vi "Dashboard Main.vi"() -> ()   [LabVIEW 2016]
uses:
  <vilib>/Utility/miscctls.llb/LVRowAndColumnTypeDef.ctl
  <vilib>/event_ctls.llb/eventvkey.ctl
  <vilib>/Rock Robotics/Network Tables/NT Read Numeric Array.vi
  Global 1.vi
  <vilib>/Rock Robotics/WPI/Dashboard/WPI_DashboardLogging Global.vi
  <vilib>/Rock Robotics/Network Tables/NT Read Boolean.vi
  <vilib>/Rock Robotics/Network Tables/NT Write Numeric Array.vi
panel:
  in  "TCP":refnum<k5>
  in  "Camera Settings Right":T1={"Frame Rate"=30, "Compression"=30, "Size"=1, "DB Camera Config"=FALSE} {"Frame Rate" scale=1.0..30.0; "Compression" scale=100.0..-1.0; "Size" items=["640x480", "320x240", "160x120"]}
  in  "Camera Name Right":string(combo)="No Camera Selection"
  out "Camera Info":cluster{"Mbps LED":bool, "Mbps":dbl, "fps":dbl} {"fps" format="%#.1g"; "Mbps" format="%#.1g"}
  in  "Camera Settings":T1={"Frame Rate"=30, "Compression"=30, "Size"=1, "DB Camera Config"=FALSE} {"Frame Rate" scale=1.0..30.0; "Compression" scale=100.0..-1.0; "Size" items=["640x480", "320x240", "160x120"]}
  in  "TCP":refnum<k5>
  in  "Rec Mode":enum32{"Stop", "Record", "Playback"}(radio)
  out "Robot IP":string
  out "Image Message":string="Timeout in Camera Communications"
  in  "Dashboard Tab":T2(tab)
  out "Boolean":bool
  in  "LockShooter":bool
  out "FrontShooter":dbl
  out "RearShooter":dbl
  in  "Select Auto":string(combo)="Select Autonomous ..."
  out "NT Connection":bool
  out "MotorChart R":cluster{"Numeric":dbl, "Numeric":dbl}(graph)
  out "MotorChart L":cluster{"Numeric":dbl, "Numeric":dbl}(graph)
  out "MotorSliders R":cluster{"MotorSlide1":dbl, "MotorSlide2":dbl} {"MotorSlide2" scale=-1.0..1.0 scale format="%#_2e"; "MotorSlide1" scale=-1.0..1.0 scale format="%#_2e"}
  out "MotorSliders L":cluster{"MotorSlide1":dbl, "MotorSlide2":dbl} {"MotorSlide2" scale=-1.0..1.0 scale format="%#_2e"; "MotorSlide1" scale=-1.0..1.0 scale format="%#_2e"}
  out "Gyro":dbl(knob) scale=0.0..360.0
  out "JS1 Z":dbl(slide) scale=-1.0..1.0 scale format="%#_2e"
  out "JS1 Graph":cluster{"X":dbl, "Y":dbl}[](graph)
  out "JS1 Buttons":T3
  out "JS2 Z":dbl(slide) scale=-1.0..1.0 scale format="%#_2e"
  out "JS2 Graph":cluster{"X":dbl, "Y":dbl}[](graph)
  out "JS2 Buttons":T3
  out "Mode":T4(ring)=enum."Auto Disabled"
  out "Camera Image Right":T5(plugin-control)
  in  "DB/String 9":string
  in  "DB/String 8":string
  in  "DB/String 7":string
  in  "DB/String 6":string
  in  "DB/String 5":string
  in  "DB/String 4":string
  in  "DB/String 3":string
  in  "DB/String 2":string
  in  "DB/String 1":string
  in  "DB/String 0":string
  in  "DB/Slider 0":dbl(slide) scale=0.0..5.0
  in  "DB/Slider 1":dbl(slide) scale=0.0..5.0
  in  "DB/Slider 2":dbl(slide) scale=0.0..5.0
  in  "DB/Slider 3":dbl(slide) scale=0.0..5.0
  out "DB/LED 3":bool
  out "DB/LED 2":bool
  out "DB/LED 1":bool
  out "DB/LED 0":bool
  in  "DB/Button 3":bool
  in  "DB/Button 2":bool
  in  "DB/Button 1":bool
  in  "DB/Button 0":bool caption="New Name"
  out "camera?":bool
  in  "dt":dbl
  out "TargetFound?":bool
  out "Yaw":dbl
  in  "AutonColor":string(combo)
  in  "AutonMode":string(combo)="DoNothing"
  out "AutonControl":string
  in  "PIDGains":dbl[](array[numeric])
  out "Countdown":sgl
  in  "Test Slider":dbl(slide) scale=0.0..100.0 scale format="%#_3g"
  in  "On/Off":bool caption="Solenoid"
  in  "Test Name":u16(ring) items=["Select the test to run..."]
  in  "Test Tree":string(tree)
  in  "Motor":cluster{"Value":dbl, "Enable":bool} {"Value" scale=-1.0..1.0 scale format="%#_3g"}
  out "Progress":T6 {"Test Progress" scale=0.0..100.0}
  in  "Rev/Fwd":cluster{"Forward":bool, "Reverse":bool}
  in  "Test Ring":u16(ring) items=["Monochrome", "Color"]
  out "Cmd Status":string
  in  "Execute Command":bool
  in  "Command Params":string[][](table)
  in  "Command Selection":i32(listbox)
  in  "CheckList":i32(listbox)
  out "Tree":string(tree)
  out "Camera Image":T5(plugin-control)
  out "Background":bool
  in  "Camera Name":string(combo)="No Camera Selection"
  # "HW"
  # "HW"
  # "Joysticks"
  # "Drive Motors"
  # "Front"
  # "Right"
  # "Left"
  # "Back"
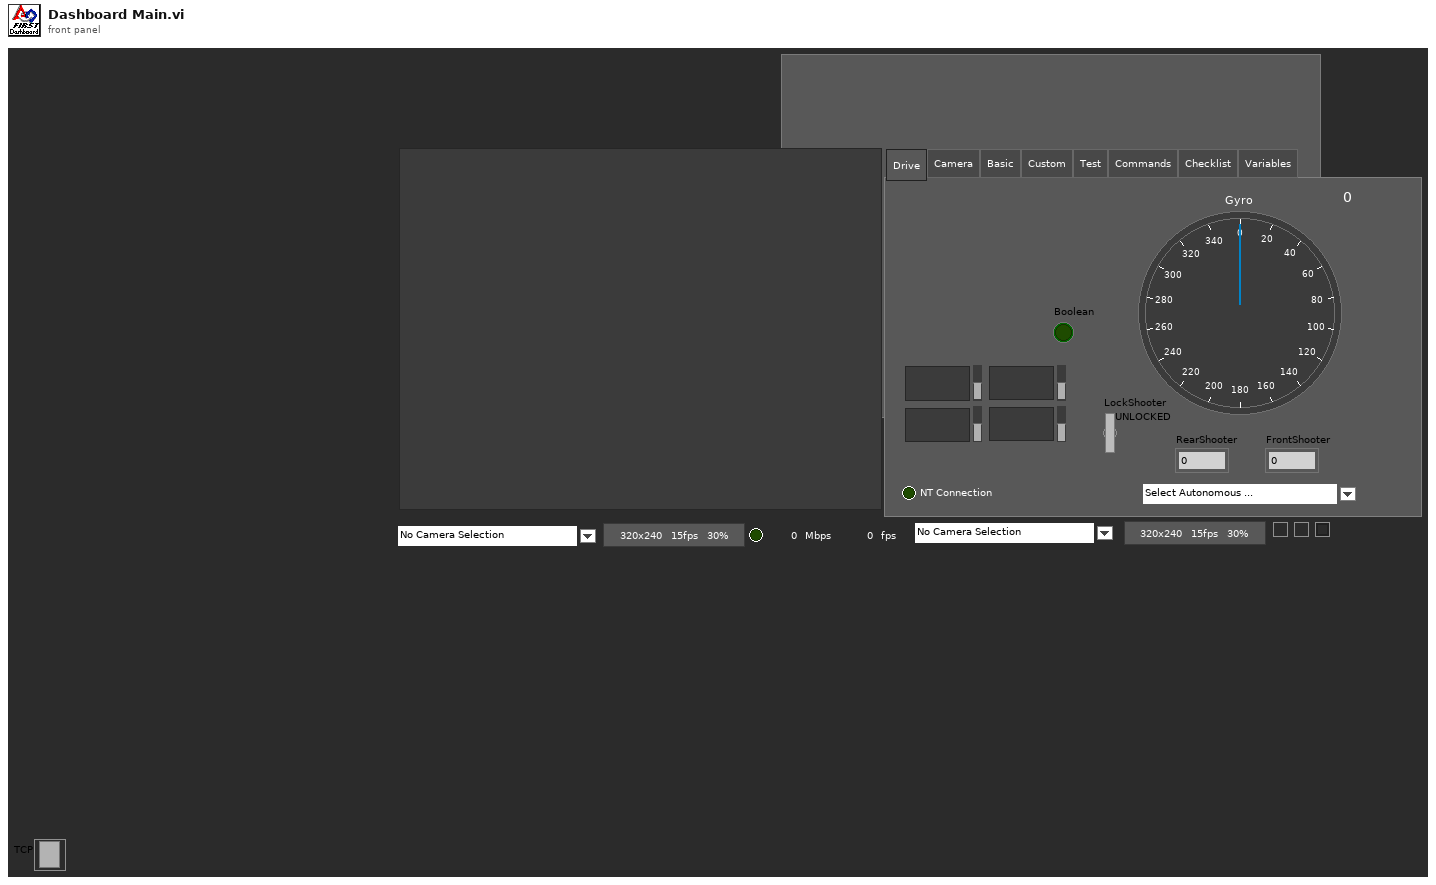
[diagram p1: front panel]
types:
  T1 = cluster{"Frame Rate":i32, "Compression":i32, "Size":u16, "DB Camera Config":bool}
  T2 = enum32{"Drive", "Camera", "Basic", "Custom", "Test", "Commands", "Checklist", "Variables"}
  T3 = cluster{bool, bool, bool, bool, bool, bool, bool, bool, bool, bool, bool, bool}
  T4 = enum8{"Tele-Op Disabled", "Tele-Op Enabled", "Auto Disabled", "Auto Enabled", "Test Disabled", "Test Enabled", "Disconnected", "No Code", "E-Stop"}
  T5 = typedef "IMAQ Image.ctl" = refnum<image>
  T6 = cluster{"Test Progress":u8, "Test Progress Text":string}
  T7 = typedef "Image Type" = u32
  T8 = cluster{"IDs":cluster{"RPC field ID":u16, "Unique ID":u16}, "String":string}
  T9 = enum32{"Drive", "Basic", "Custom", "Test", "Checklist", "Variables"}
  T10 = cluster{"Camera Image":refnum<vi>, "Dashboard Tab":refnum<vi>, "Background":refnum<vi>, "Rec Mode":refnum<vi>, "Test Slider":refnum<vi>, "On/Off ":refnum<vi>, "Test Ring":refnum<vi>, "Rev/Fwd":refnum<vi>, "Test Name":refnum<vi>, "Motor":refnum<vi>, "Progress":refnum<vi>, "CheckList":refnum<vi>, "Tree":refnum<vi>, "Test Tree":refnum<vi>, "Command Params":refnum<vi>, "Command Selection":refnum<vi>, "Execute Command":refnum<vi>, "Cmd Status":refnum<vi>, "Camera Settings":refnum<vi>, "Camera Name":refnum<vi>, "Camera Info":refnum<vi>, "Camera Settings Right":refnum<vi>, "Camera Name Right":refnum<vi>, "Camera Image Right":refnum<vi>}
  T11 = cluster{"Control Bits":cluster{"TestMode":bool, "Autonomous":bool, "Enabled":bool, "FMS Present":bool, bool, bool, bool, "E-Stop":bool}, "Team Station ":u8, "Countdown":sgl, "Joystick Values":cluster{"Axes":dbl[], "Buttons":bool[], "POVs":i16[]}[]}
  T12 = cluster{"Axes":dbl[], "Buttons":bool[], "POVs":i16[]}[]
  T13 = cluster{"Axes":dbl[], "Buttons":bool[], "POVs":i16[]}
  T14 = cluster{"Error Strings":string, "Disable Counts":cluster{u16, u16}, "Rail Faults":cluster{u16, u16, u16}, "Robot IP":string, "DB Mode":u8, "Event Info":cluster{"Name":string, "Type":u8, "Number":u16, "Replay":u8}}
  T15 = cluster{"Storage":cluster{"Disk Free":u64, "RAM Block":u32, "RAM free":u32}, "CPU Utilization":cluster{"CPU % ISR":sgl, "CPU % Time Crit":sgl, "CPU % Timed Str":sgl, "CPU % High":sgl, "CPU % Above":sgl, "CPU % Normal":sgl, "CPU % Low":sgl}, "CAN":cluster{"% Bus Utilization":sgl, "Bus Off Cnt":u32, "TX_FIFO Full Cnt":u32, "Receive Error Cnt":u8, "Transmit Error Cnt":u8}, "HID":cluster{"HID Outputs":u32, "Rumble Low":u16, "Rumble High":u16}[]}
  T16 = cluster{"Status bits":cluster{"Test Mode":bool, "Autonomous":bool, "Enabled":bool, "Code Start":bool, "Brownout":bool, "Reserved 2":bool, "Reserved 3":bool, "E-Stop":bool}, "Code Trace":cluster{"Disabled":bool, "TeleOp":bool, "Auto":bool, "Test":bool}, "Controller Type":enum16{"unknown", "cRIO", "roboRio"}, "Code?":enum16{"unknown", "noCode", "code"}, "Battery V":dbl}
  T17 = cluster{"Buttons[0]":bool, "Buttons[1]":bool, "Buttons[2]":bool, "Buttons[3]":bool, "Buttons[4]":bool, "Buttons[5]":bool, "Buttons[6]":bool, "Buttons[7]":bool, "Buttons[8]":bool, "Buttons[9]":bool, "Buttons[10]":bool, "Buttons[11]":bool}
  T18 = cluster{"Operation":enum16{"Update", "Clear"}, "Color Box":u32}[]
  T19 = typedef "eventvkey.ctl" = enum16{"ASCII", "Enter", "Return", "Shift", "Ctrl", "Alt", "Cmd", "Opt", "Caps", "NumLock", "Clear", "Break", "Up", "Down", "Left", "Right", "Insert", "Delete", "Home", "End", "PageUp", "PageDown", "Escape", "Help", "Pause", "ScrollLock", "F1", "F2", "F3", "F4", "F5", "F6", "F7", "F8", "F9", "F10", "F11", "F12", "F13", "F14", "F15", "F16", "F17", "F18", "F19", "F20", "F21", "F22", "F23", "F24", "Play", "VolumeUp", "VolumeDown", "Mute", "Two Byte Char"}
  T20 = cluster{"Image Size":bool, "Image Type":bool, "Pixel Value":bool, "ROI Information":bool, "Zoom Factor":bool}
  T21 = cluster{"Operation":enum16{"Update", "Clear"}, "Color Box":u32}
  T22 = typedef "LVRowAndColumnTypeDef.ctl" = cluster{"Row":i32, "Column":i32}
  T23 = cluster{"Shift":bool, "Ctrl":bool, "Alt":bool, "Cmd":bool, "Opt":bool}
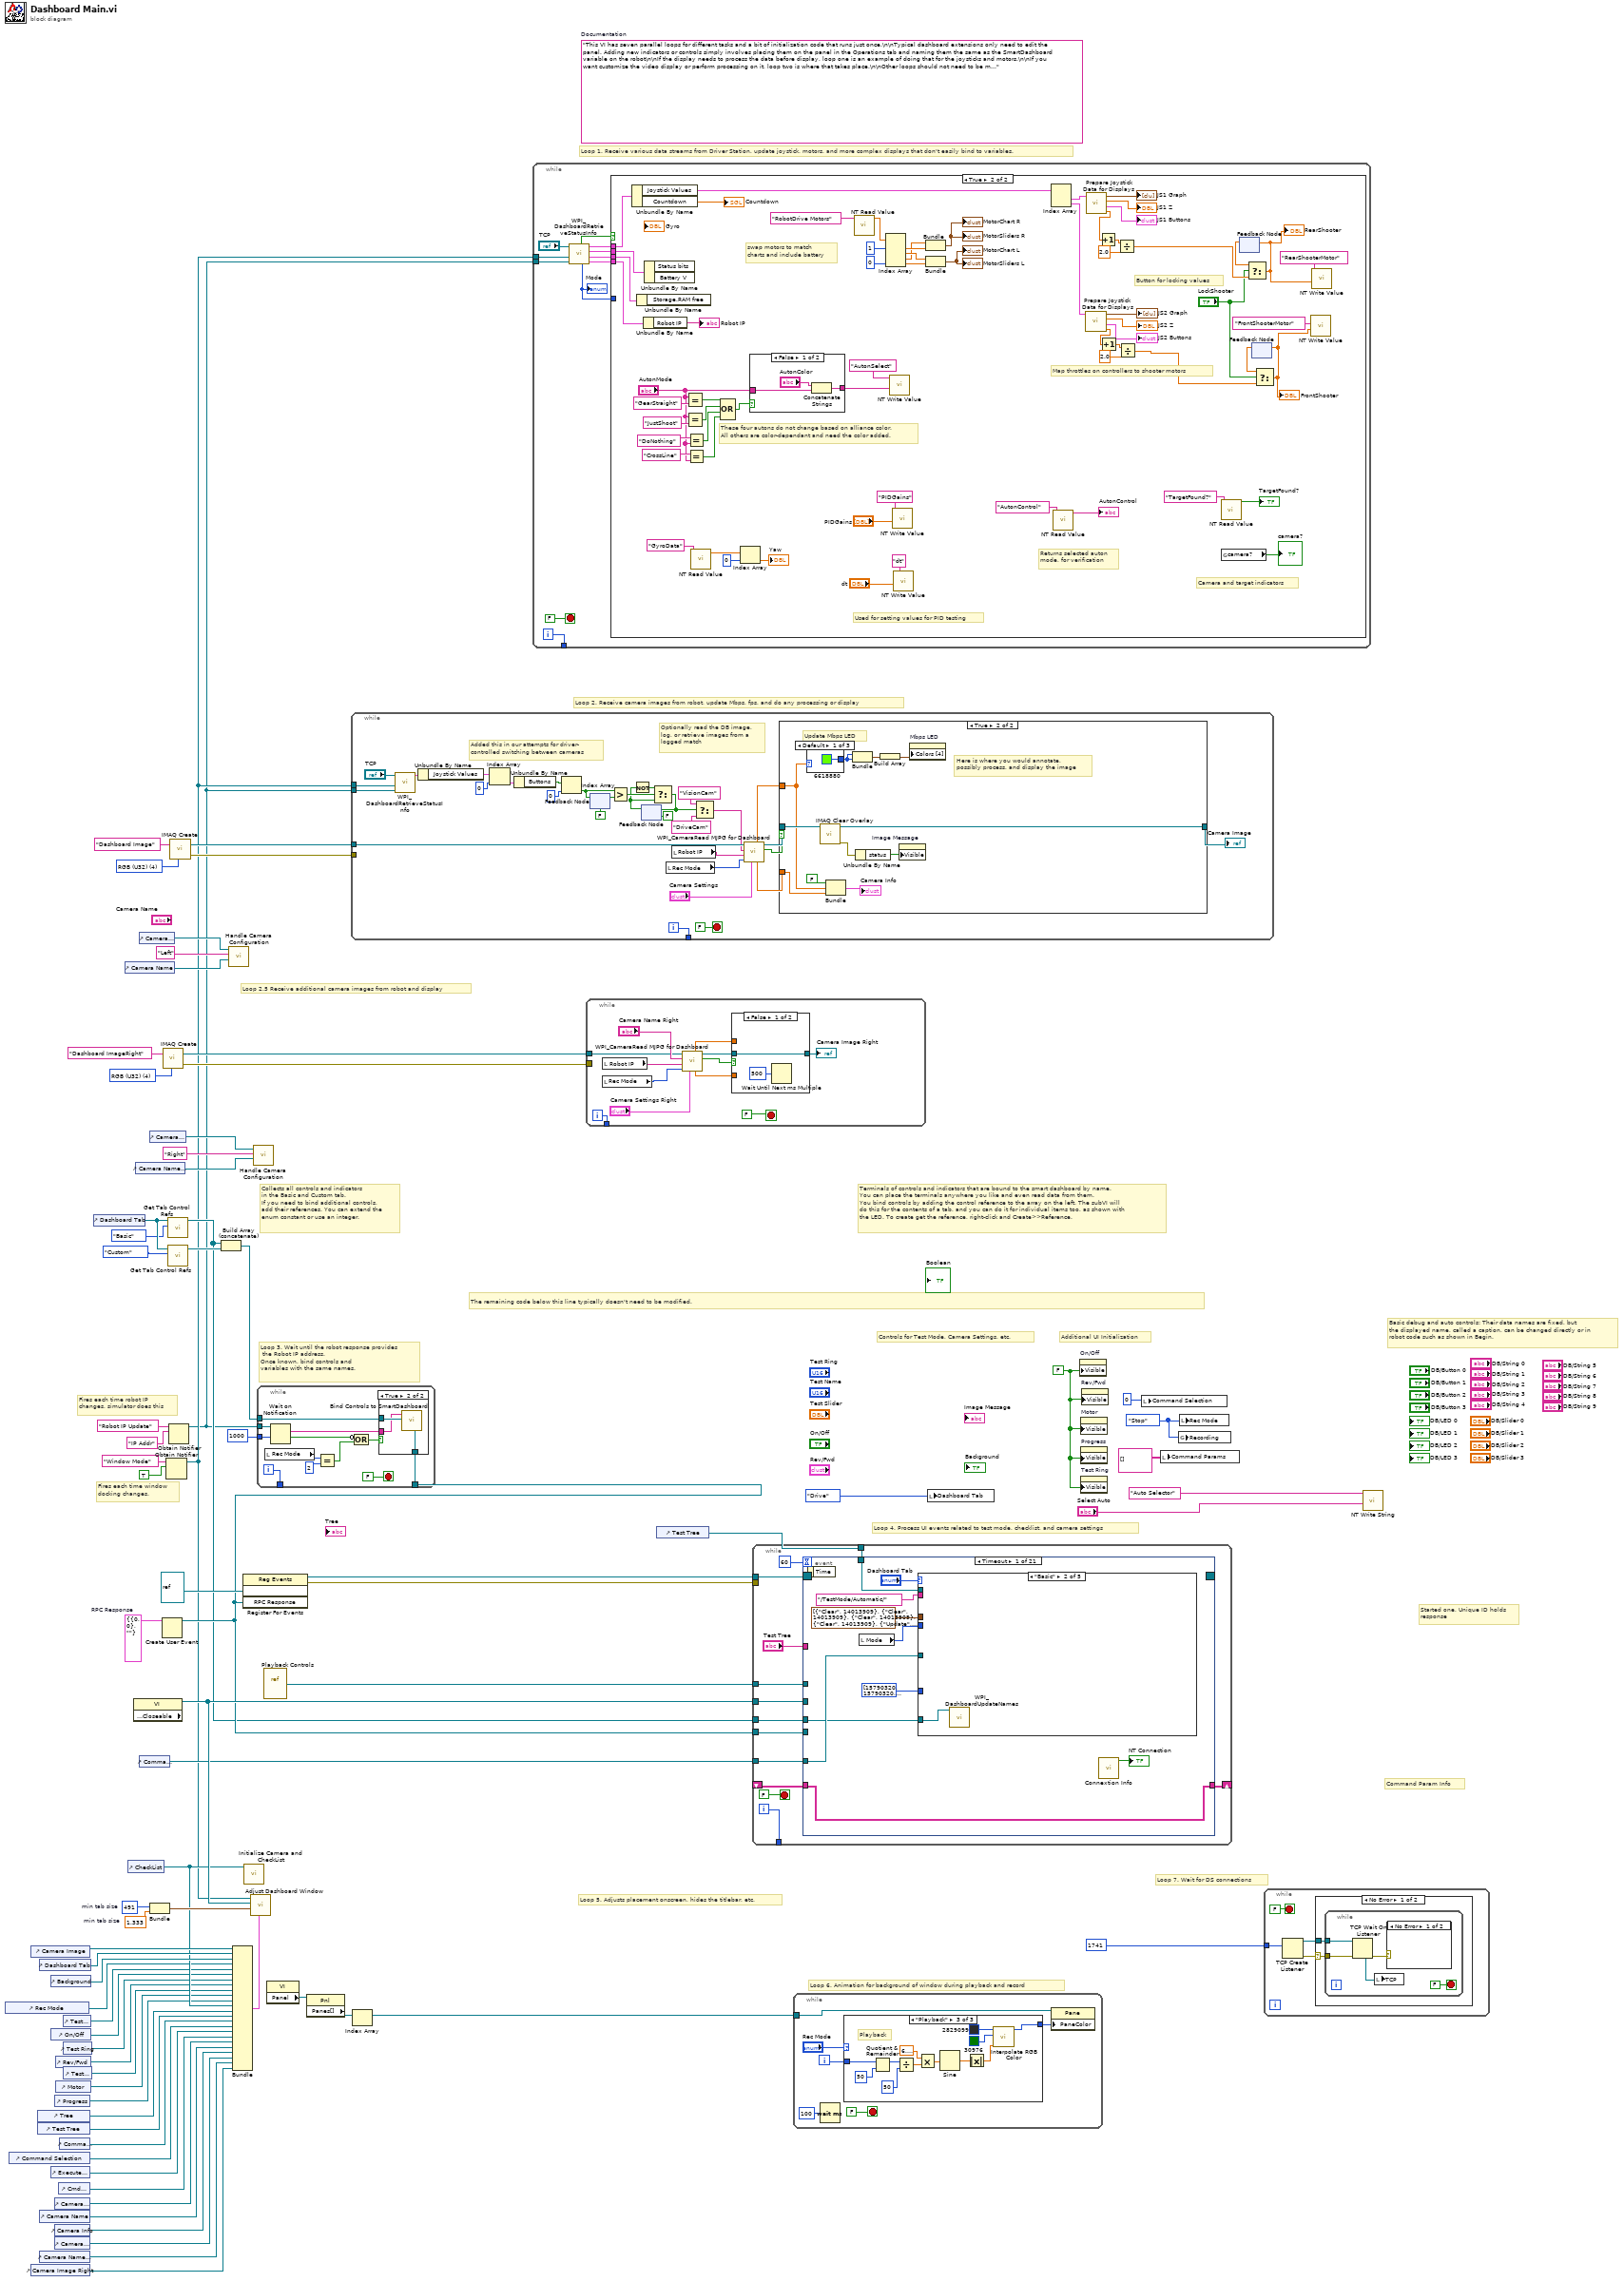
[diagram p0: block diagram]
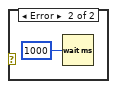
[diagram p3: hidden frame]
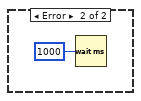
[diagram p4: hidden frame]
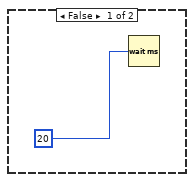
[diagram p5: hidden frame]
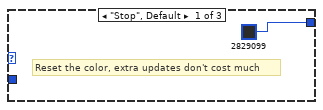
[diagram p7: hidden frame]
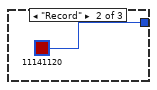
[diagram p8: hidden frame]
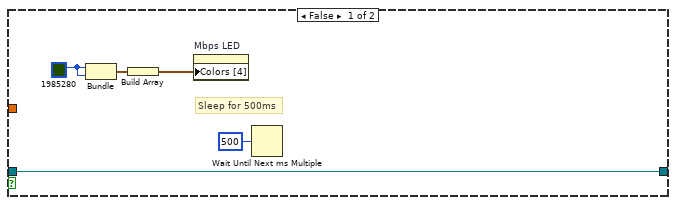
[diagram p10: hidden frame]
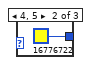
[diagram p11: hidden frame]
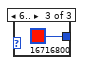
[diagram p12: hidden frame]
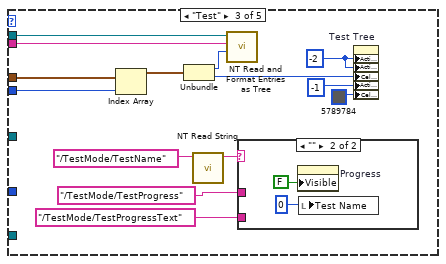
[diagram p14: hidden frame]
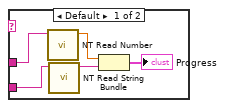
[diagram p15: hidden frame]
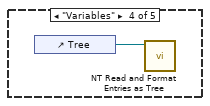
[diagram p16: hidden frame]
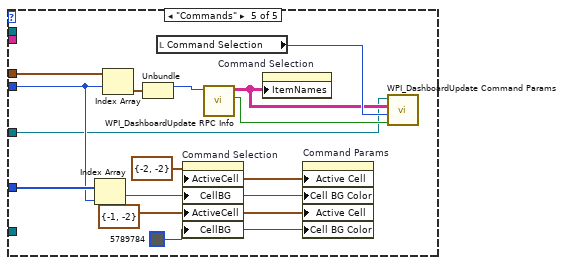
[diagram p17: hidden frame]
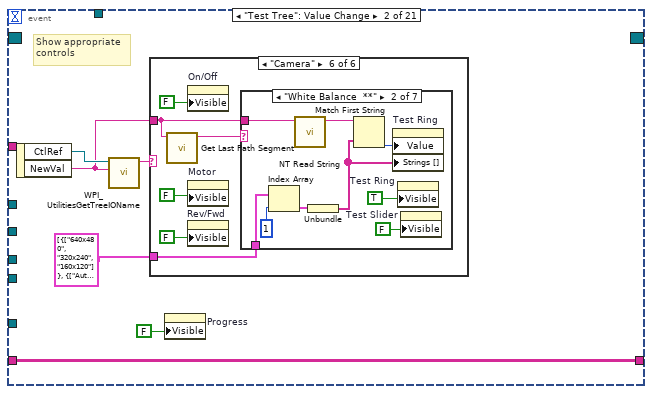
[diagram p18: hidden frame]
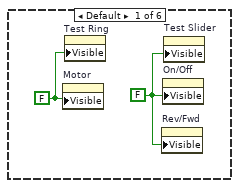
[diagram p19: hidden frame]
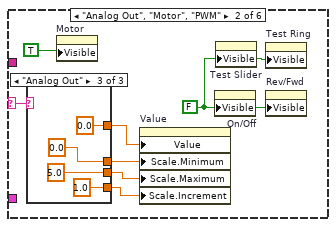
[diagram p20: hidden frame]
diagram:
  w12 = T7 4 items=["Grayscale (U8)", "Grayscale (I16)", "Grayscale (SGL)", "Complex (CSG)", "RGB (U32)", "HSL (U32)", "RGB (U64)"] ("Image Type")
  w28 = T8 {"IDs"={"RPC field ID"=0, "Unique ID"=0}, "String"=""}  # RPC Response
  w51 = 491  # min tab size
  w50 = 1.333  # min tab size
  w58 = enum32{"Stop", "Record", "Playback"}."Stop" ("Rec Mode")
  w33 = FALSE ("Visible")
  (unwired) "This VI has seven parallel loops for different tasks and a bit of initialization code that runs just once.\n\nTypical dashboard extensions only need to edit the panel. Adding new indicators or controls simply involves placing them on the panel in the Operations tab and naming them the same as the SmartDashboard variable on the robot\n\nIf the display needs to process the data before display, loop one is an example of doing that for the joysticks and motors.\n\nIf you want customize the video display or perform processing on it, loop two is where that takes place.\n\nOther loops should not need to be modified. They are pretty standard, and document the task they perform."  # Documentation
  w75 = T7 4 items=["Grayscale (U8)", "Grayscale (I16)", "Grayscale (SGL)", "Complex (CSG)", "RGB (U32)", "HSL (U32)", "RGB (U64)"] ("Image Type")
  # "Loop 2.5 Receive additional camera images from robot and display"
  # "Command Param Info"
  # "Started one, Unique ID holds\nresponse"
  # "Loop 7. Wait for DS connections"
  # "Basic debug and auto controls: Their data names are fixed, but\nthe displayed name, called a caption, can be changed directly or in\nrobot code such as shown in Begin."
  # "Controls for Test Mode, Camera Settings, etc."
  # "Additional UI Initialization"
  # "Loop 6. Animation for background of window during playback and record"
  # "Fires each time robot IP\nchanges, simulator does this"
  # "Fires each time window\ndocking changes."
  # "Collects all controls and indicators\nin the Basic and Custom tab.\nIf you need to bind additional controls,\nadd their references. You can extend the\nenum constant or use an integer."
  # "The remaining code below this line typically doesn't need to be modified."
  # "Loop 4. Process UI events related to test mode, checklist, and camera settings"
  # "Terminals of controls and indicators that are bound to the smart dashboard by name.\nYou can place the terminals anywhere you like and even read data from them.\nYou bind controls by adding the control reference to the array on the left. The subVI will\ndo this for the contents of a tab, and you can do it for individual items too, as shown with\nthe LED. To create get the reference, right-click and Create>>Reference."
  # "Loop 3. Wait until the robot response provides\n the Robot IP address.\nOnce known, bind controls and\nvariables with the same names."
  # "Loop 5. Adjusts placement onscreen, hides the titlebar, etc."
  # "Loop 1. Receive various data streams from Driver Station, update joystick, motors, and more complex displays that don't easily bind to variables."
  # "Loop 2. Receive camera images from robot, update Mbps, fps, and do any processing or display"
  n1 = control-ref of="Rec Mode"() -> (w39:refnum<vi>)
  n2 = control-ref of="Command Selection"() -> (w27:refnum<vi>)
  n3 = control-ref of="Camera Image Right"() -> (w3:refnum<vi>)
  n4 = control-ref of="Camera Image"() -> (w53:refnum<vi>)
  n5 = control-ref of="Tree"() -> (w43:refnum<vi>)
  n6 = control-ref of="Test Tree"() -> (w42:refnum<vi>)
  n7 = control-ref of="Dashboard Tab"() -> (w52:refnum<vi>)
  n8 = control-ref of="Camera Name"() -> (w18:refnum<vi>)
  n9 = control-ref of="Camera Name Right"() -> (w4:refnum<vi>)
  n10 = control-ref of="Execute Command"() -> (w29:refnum<vi>)
  n11 = control-ref of="Background"() -> (w48:refnum<vi>)
  n12 = control-ref of="On/Off"() -> (w37:refnum<vi>)
  n13 = control-ref of="Progress"() -> (w34:refnum<vi>)
  n14 = control-ref of="Camera Settings"() -> (w19:refnum<vi>)
  n15 = control-ref of="Camera Info"() -> (w17:refnum<vi>)
  n16 = control-ref of="Camera Settings Right"() -> (w5:refnum<vi>)
  n17 = control-ref of="Rev/Fwd"() -> (w35:refnum<vi>)
  n18 = control-ref of="Motor"() -> (w40:refnum<vi>)
  n19 = control-ref of="Cmd Status"() -> (w23:refnum<vi>)
  n20 = control-ref of="Command Params"() -> (w30:refnum<vi>)
  n21 = control-ref of="Test Slider"() -> (w38:refnum<vi>)
  n22 = control-ref of="Test Ring"() -> (w36:refnum<vi>)
  n23 = control-ref of="Test Name"() -> (w41:refnum<vi>)
  n24 = control-ref of="Dashboard Tab"() -> (w56:refnum<vi>)
  n25 = control-ref of="Camera Name"() -> (w20:refnum<vi>)
  n26 = control-ref of="CheckList"() -> (w44:refnum<vi>)
  n27 = property class="VI" props=["Front Panel.Closeable"]() -> (reference out=w57:refnum<vi>)  [unwired: 2 in, 2 out]
  n28 = control-ref of="Camera Name Right"() -> (w8:refnum<vi>)
  n29 = control-ref of="Camera Settings"() -> (w21:refnum<vi>)
  n30 = control-ref of="Command Params"() -> (w22:refnum<vi>)
  n31 = control-ref of="Camera Settings Right"() -> (w9:refnum<vi>)
  n32 = Bundle("min tab size"=w51, "min tab size"=w50) -> (w49:cluster{"min tab size":i32, "min tab size":dbl})  [unwired: 1 in]
  n33 = Create User Event(user event datatype=w28) -> (user event=w24:refnum<user-event>)  [unwired: 1 in, 1 out]
  n34 = call "IMAQ Create"("Image Name"="Dashboard ImageRight", "Image Type"=w12) -> ("New Image"=w11:T5, "error out"=w10:errorcluster)  [unwired: 2 in, 1 out]
  n35 = Obtain Notifier(name (unnamed)="Window Mode", notification data type=TRUE) -> (notifier out=w2:refnum<notifier>)  [unwired: 2 in, 2 out]
  n36 = call <vilib>:"Get Tab Control Refs.vi"("Page Index"=T9."Basic" ("Dashboard Tab"), "TabControl in"=w56) -> ("ControlsOnPage"=w16:refnum<vi>[])  [unwired: 9 in]
  n37 = call <vilib>:"Get Tab Control Refs.vi"("Page Index"=T9."Custom" ("Dashboard Tab"), "TabControl in"=w56) -> ("ControlsOnPage"=w55:refnum<vi>[])  [unwired: 9 in]
  n38 = Obtain Notifier(name (unnamed)="Robot IP Update", notification data type="IP Addr" ("name (unnamed)")) -> (notifier out=w1:refnum<notifier>)  [unwired: 2 in, 2 out]
  n39 = call "IMAQ Create"("Image Name"="Dashboard Image", "Image Type"=w75) -> ("New Image"=w73:T5, "error out"=w72:errorcluster)  [unwired: 2 in, 1 out]
  n40 = Build Array (concatenate)(w16, w55) -> (w54:refnum<vi>[])
  n41 = call "Handle Camera Configuration.vi"("CameraNameRef"=w20, "Camera File Name"="Left", "ClusterRef"=w21) -> ()  [unwired: 9 in]
  n42 = Bundle("Camera Image"=w53, "Dashboard Tab"=w52, "Background"=w48, "Rec Mode"=w39, "Test Slider"=w38, "On/Off"=w37, "Test Ring"=w36, "Rev/Fwd"=w35, "Test Name"=w41, "Motor"=w40, "Progress"=w34, "CheckList"=w44, "Tree"=w43, "Test Tree"=w42, "Command Params"=w30, "Command Selection"=w27, "Execute Command"=w29, "Cmd Status"=w23, "Camera Settings"=w19, "Camera Name"=w18, "Camera Info"=w17, "Camera Settings Right"=w5, "Camera Name Right"=w4, "Camera Image Right"=w3) -> (w45:T10)  [unwired: 1 in]
  n43 = register-events(refnum<vi> refnum, w24) -> (reference out=w62:refnum<event-registration>, error out=w61:errorcluster)  [unwired: 2 in]
  n44 = call "Initialize Camera and CheckList.vi"("ListBox in"=w44) -> ()  [unwired: 11 in]
  n45 = call "Adjust Dashboard Window.vi"("Sizing Refnums"=w45, "Size Constraints"=w49, "VI"=w57, "WIn Mode"=w2) -> ()  [unwired: 8 in]
  n46 = call "Handle Camera Configuration.vi"("CameraNameRef"=w8, "Camera File Name"="Right", "ClusterRef"=w9) -> ()  [unwired: 9 in]
  n47 = while {
    tunnel: w54 -> [w87]
    tunnel: w1 -> [w85]
    tunnel: [w83] -> _
    tunnel: u32 1000 ("milliseconds to wait") -> [w82]
    tunnel: w24 -> [w76]
    i -> [w83]
    stop <- FALSE stop-if-true
    n48 = local read "Rec Mode"() -> (w78:enum32{"Stop", "Record", "Playback"})
    n49 = Wait on Notification(notifier=w85, timeout in ms (-1)=w82) -> (notification=w84:string, timed out?=w80:bool)  [unwired: 2 in, 2 out]
    n50 = Equal?(x=w78, y=u16 2 ("Rec Mode")) -> (x = y?=w79:bool)
    n51 = Compound Arithmetic op=OR(invert w80, w79) -> (w81:bool)
    n52 = case shown="True" w81 {
      tunnel: w87 -> [_ w90]
      tunnel: w84 -> [_ w89]
      tunnel: w76 -> [_ w88]
      frame False {
      }
      frame True {
        n53 = call <vilib>:"Bind Controls to SmartDashboard.vi"("RPC ref"=w88, "Bound Control Refs"=w90, "Server IP Address"=w89) -> ()  [unwired: 9 in]
      }
    }
  }
  n54 = vi-ref "Playback Controls.vi"() -> (w63:refnum<vi>)
  n55 = property class="VI"() -> ("Panel"=w65:refnum<vi>)  [unwired: 2 in, 2 out]
  n56 = property class="Pnl"(reference=w65) -> ("Panes[]"=w66:refnum<vi>[])  [unwired: 1 in, 2 out]
  n57 = while {
    tunnel: w73 -> [w119]
    tunnel: w72 -> [_]
    tunnel: [w120] -> _
    tunnel: w2 -> [w109]
    tunnel: w1 -> [w108]
    i -> [w120]
    stop <- FALSE stop-if-true
    # "Added this in our attempts for driver-\ncontrolled switching between cameras"
    # "Optionally read the DB image,\nlog, or retrieve images from a\nlogged match"
    n58 = call <vilib>:"WPI_DashboardRetrieveStatusInfo.vi"("Binding Refnum"=w108, "Window Mode Notifier"=w109, "TCP Cnx"="TCP") -> ("Control Info"=w107:T11)  [unwired: 3 in, 5 out]
    n59 = Unbundle By Name(w107) -> ("Joystick Values"=w106:T12)
    n60 = Index Array(array=w106, index=0) -> (element=w104:T13)
    n61 = Unbundle By Name(w104) -> ("Buttons"=w103:bool[])
    n62 = Index Array(array=w103, index=0) -> (element=w100:bool)
    n63 = feedback-in #1(w100) -> ()
    n64 = feedback #1(FALSE) -> (w101:bool)
    n65 = Greater?(x=w100, y=w101) -> (0:w98:bool)
    n66 = feedback #2(FALSE) -> (w95:bool)
    n67 = Not(x=w95) -> (.not. x?=w96:bool)
    n68 = Select(t=w96, s=w98, f=w95) -> (s? t:f=w93:bool)
    n69 = feedback-in #2(w93) -> ()
    n70 = local read "Rec Mode"() -> (w115:enum32{"Stop", "Record", "Playback"})
    n71 = local read "Robot IP"() -> (w114:string)
    n72 = Select(t="VisionCam", s=w93, f="DriveCam") -> (s? t:f=w91:string)
    n73 = call <vilib>:"WPI_CameraRead MJPG for Dashboard.vi"("Camera Settings"="Camera Settings", "Rec Mode"=w115, "Robot IP"=w114, "Camera Name"=w91, "Refnum in"=w119) -> ("Active"=w117:bool, "Refnum out"=w118:T5, "FPS"=w116:dbl, "Bandwidth (Mbps)"=w113:dbl)  [unwired: 3 in]
    n74 = case shown="True" w117 {
      tunnel: w118 -> [w122 w133]
      tunnel: w113 -> [_ w130]
      tunnel: w116 -> [_ w131]
      tunnel: [w122 w127] -> w111
      frame False {
        w124 = u32 1985280 ("Color Box")
        # "Sleep for 500ms"
        n75 = Bundle("Color Box"=w124, "Color Box"=w124) -> (w125:cluster{"Color Box":u32, "Color Box":u32})  [unwired: 1 out]
        n76 = Build Array(w125) -> (w123:cluster{"Color Box":u32, "Color Box":u32}[])
        n77 = property on="Mbps LED" class="Bool (strict)"("Colors [4]"=w123) -> ()  [unwired: 2 in, 2 out]
        n78 = Wait Until Next ms Multiple(millisecond multiple=u32 500) -> ()  [unwired: 1 out]
      }
      frame True {
        # "Here is where you would annotate,\npossibly process, and display the image"
        # "Update Mbps LED"
        n79 = case shown="Default" w130 {
          tunnel: [u32 6618880 ("Color Box") u32 16776722 ("Color Box") u32 16716800 ("Color Box")] -> w134
          frame Default {
          }
          frame 4, 5 {
          }
          frame 6.. {
          }
        }
        n80 = call "IMAQ Clear Overlay"("Image"=w133) -> ("error out"=w136:errorcluster, "Image Out"=w127:T5)  [unwired: 2 in, 7 out]
        n81 = Bundle(FALSE, "Bandwidth (Mbps)"=w130, "FPS"=w131) -> (→"Camera Info":cluster{bool, "Bandwidth (Mbps)":dbl, "FPS":dbl})  [unwired: 1 in]
        n82 = Bundle("Color Box"=w134, "Color Box"=w134) -> (w135:cluster{"Color Box":u32, "Color Box":u32})  [unwired: 1 out]
        n83 = Unbundle By Name(w136) -> ("status"=w137:bool)
        n84 = Build Array(w135) -> (w132:cluster{"Color Box":u32, "Color Box":u32}[])
        n85 = property on="Image Message" class="Str"("Visible"=w137) -> ()  [unwired: 2 in, 2 out]
        n86 = property on="Mbps LED" class="Bool (strict)"("Colors [4]"=w132) -> ()  [unwired: 2 in, 2 out]
      }
    }
    "Camera Image" <- w111
  }
  n87 = Index Array(array=w66) -> (element=w64:refnum<vi>)  [unwired: 1 in]
  n88 = while {
    tunnel: [w150] -> _
    tunnel: w1 -> [w144]
    tunnel: w2 -> [w141]
    i -> [w150]
    stop <- FALSE stop-if-true
    n89 = call <vilib>:"WPI_DashboardRetrieveStatusInfo.vi"("Binding Refnum"=w144, "Window Mode Notifier"=w141, "TCP Cnx"="TCP") -> ("Power and Errors"=w145:T14, "Robot Metrics"=w148:T15, "Status Info"=w149:T16, "Control Info"=w146:T11, "Robot Mode"=w143:T4, "Process?"=w147:bool)  [unwired: 3 in]
    "Mode" <- w143
    n90 = case shown="True" w147 {
      tunnel: w149 -> [_ w217]
      tunnel: w148 -> [_ w216]
      tunnel: w146 -> [_ w215]
      tunnel: w145 -> [_ w214]
      tunnel: w143 -> [_ _]
      frame False {
        n91 = Wait (ms)(milliseconds to wait=u32 20) -> ()  [unwired: 1 out]
      }
      frame True {
        # "Returns selected auton\nmode, for verification"
        # "These four autons do not change based on alliance color.\nAll others are color-dependant and need the color added."
        # "Used for setting values for PID testing"
        # "Camera and target indicators"
        # "Button for locking values"
        # "Map throttles on controllers to shooter motors"
        # "swap motors to match\ncharts and include battery"
        n92 = Unbundle By Name(w215) -> ("Joystick Values"=w205:T12, "Countdown"=→"Countdown":sgl)
        n93 = Unbundle By Name(w216) -> ()  [unwired: 1 out]
        n94 = Unbundle By Name(w214) -> ("Robot IP"=→"Robot IP":string)
        n95 = Unbundle By Name(w217) -> ()  [unwired: 2 out]
        n96 = Equal?(x="AutonMode", y="GearStraight") -> (x = y?=w175:bool)
        n97 = Equal?(x="AutonMode", y="JustShoot") -> (x = y?=w174:bool)
        n98 = Equal?(x="DoNothing", y="AutonMode") -> (x = y?=w172:bool)
        n99 = Equal?(x="CrossLine", y="AutonMode") -> (x = y?=w169:bool)
        n100 = call-poly <vilib>:"NT Read Value.vi"("Name"="GyroData") -> ("Numeric Array"=w186:dbl[])  [unwired: 9 in, 1 out]
        n101 = Compound Arithmetic op=OR(w175, w174, w172, w169) -> (w173:bool)
        n102 = Index Array(array=w186, index=0) -> (element=→"Yaw":dbl)
        n103 = case shown="False" w173 {
          tunnel: [w220 w221] -> w193
          tunnel: "AutonMode" -> [w218 w221]
          frame False {
            n104 = Concatenate Strings("AutonColor", w218) -> (w220:string)
          }
          frame True, Default {
          }
        }
        n105 = call-poly <vilib>:"NT Read Value.vi"("Name"="RobotDrive Motors") -> ("Numeric Array"=w195:dbl[])  [unwired: 9 in, 1 out]
        n106 = Index Array(array=w195, index #1=1, index #4=0) -> (element #1=w209:dbl, element #2=w210:dbl, element #3=w208:dbl, element #4=w213:dbl)  [unwired: 2 in]
        n107 = call-poly <vilib>:"NT Write Value.vi"("String"=w193, "Name"="AutonSelect") -> ()  [unwired: 9 in, 1 out]
        n108 = call-poly <vilib>:"NT Write Value.vi"("Numeric Array"="PIDGains", "Name"="PIDGains") -> ()  [unwired: 9 in, 1 out]
        n109 = call-poly <vilib>:"NT Write Value.vi"("Numeric"="dt", "Name"="dt") -> ()  [unwired: 9 in, 1 out]
        n110 = Bundle("Numeric"=w208, "Numeric"=w209) -> (→"MotorChart R" →"MotorSliders R":cluster{"Numeric":dbl, "Numeric":dbl})  [unwired: 1 in]
        n111 = Bundle("Numeric"=w210, "Numeric"=w213) -> (→"MotorChart L" →"MotorSliders L":cluster{"Numeric":dbl, "Numeric":dbl})  [unwired: 1 in]
        n112 = Index Array(array=w205) -> (element #1=w204:T13, element #2=w200:T13)  [unwired: 2 in]
        n113 = call-poly <vilib>:"NT Read Value.vi"("Name"="AutonControl") -> ("String"=→"AutonControl":string)  [unwired: 9 in, 1 out]
        n114 = call "Prepare Joystick Data for Displays.vi"("Joystick Values"=w200) -> ("Throttle"=w162:dbl, "Buttons"=→"JS2 Buttons":T17, "Z Axis"=→"JS2 Z":dbl, "Cartesian Data"=→"JS2 Graph":cluster{"X axis":dbl, "X axis":dbl}[])  [unwired: 7 in]
        n115 = call "Prepare Joystick Data for Displays.vi"("Joystick Values"=w204) -> ("Throttle"=w167:dbl, "Buttons"=→"JS1 Buttons":T17, "Z Axis"=→"JS1 Z":dbl, "Cartesian Data"=→"JS1 Graph":cluster{"X axis":dbl, "X axis":dbl}[])  [unwired: 7 in]
        n116 = Increment(x=w167) -> (x+1=w166:dbl)
        n117 = Increment(x=w162) -> (x+1=w163:dbl)
        n118 = Divide(x=w166, y=2.0) -> (x/y=w161:dbl)
        n119 = Divide(x=w163, y=2.0) -> (x/y=w157:dbl)
        n120 = global read "Global 1.vi" "camera?"() -> (→"camera?":bool)
        n121 = call-poly <vilib>:"NT Read Value.vi"("Name"="TargetFound?") -> ("Boolean"=→"TargetFound?":bool)  [unwired: 9 in, 1 out]
        n122 = feedback #3() -> (w160:dbl)  [unwired: 1 in]
        n123 = Select(t=w160, s="LockShooter", f=w161) -> (s? t:f=w153:dbl)
        "RearShooter" <- w153
        n124 = feedback-in #3(w153) -> ()
        n125 = feedback #4() -> (w158:dbl)  [unwired: 1 in]
        n126 = Select(t=w158, s="LockShooter", f=w157) -> (s? t:f=w155:dbl)
        "FrontShooter" <- w155
        n127 = feedback-in #4(w155) -> ()
        n128 = call-poly <vilib>:"NT Write Value.vi"("Numeric"=w155, "Name"="FrontShooterMotor") -> ()  [unwired: 9 in, 1 out]
        n129 = call-poly <vilib>:"NT Write Value.vi"("Numeric"=w153, "Name"="RearShooterMotor") -> ()  [unwired: 9 in, 1 out]
      }
    }
  }
  n130 = while {
    tunnel: w11 -> [w232]
    tunnel: w10 -> [_]
    tunnel: [w226] -> _
    i -> [w226]
    stop <- FALSE stop-if-true
    n131 = local read "Rec Mode"() -> (w230:enum32{"Stop", "Record", "Playback"})
    n132 = local read "Robot IP"() -> (w231:string)
    n133 = call <vilib>:"WPI_CameraRead MJPG for Dashboard.vi"("Camera Settings"="Camera Settings Right", "Rec Mode"=w230, "Robot IP"=w231, "Camera Name"="Camera Name Right", "Refnum in"=w232) -> ("Active"=w225:bool, "Refnum out"=w228:T5, "FPS"=w223:dbl, "Bandwidth (Mbps)"=w224:dbl)  [unwired: 3 in]
    n134 = case shown="False" w225 {
      tunnel: w228 -> [w234 w236]
      tunnel: w224 -> [_ _]
      tunnel: w223 -> [_ _]
      tunnel: [w234 w236] -> w222
      frame False {
        n135 = Wait Until Next ms Multiple(millisecond multiple=u32 500) -> ()  [unwired: 1 out]
      }
      frame True {
      }
    }
    "Camera Image Right" <- w222
  }
  n136 = control-ref of="Test Tree"() -> (w67:refnum<vi>)
  n137 = while {
    tunnel: [w246] -> _
    tunnel: w67 -> [w245]
    tunnel: w63 -> [w244]
    tunnel: w62 -> [w243]
    tunnel: w61 -> [_]
    tunnel: w57 -> [w242]
    tunnel: w24 -> [w241]
    tunnel: w22 -> [w240]
    shift-right: [w239] -> _
    shift-left: _ -> [w238]
    tunnel: w16 -> [w237]
    i -> [w246]
    stop <- FALSE stop-if-true
    n138 = event shown="[0] Timeout" {
      selector: w243 -> [_ _ _ _ _ _ _ _ _ _ _ _ _ _ _ _ _ _ _ _ _]
      dyn-events: [_ _ _ _ _ _ _ _ _ _ _ _ _ _ _ _ w502 _ _ _ _] -> _
      timeout: u32 60 ("milliseconds to wait") -> [_ _ _ _ _ _ _ _ _ _ _ _ _ _ _ _ _ _ _ _ _]
      tunnel: w245 -> [w258 _ _ _ _ _ _ _ _ _ _ _ _ _ _ _ _ _ _ _ _]
      tunnel: "Test Tree" -> [_ _ _ _ _ _ _ _ _ _ _ w469 w477 w479 w483 w491 _ _ _ _ _]
      tunnel: w244 -> [_ _ _ _ _ _ _ _ _ _ _ _ _ _ _ _ w504 _ w522 _ _]
      tunnel: w242 -> [_ _ _ _ _ _ _ _ _ _ _ _ _ _ _ _ w500 _ _ _ _]
      tunnel: w241 -> [_ _ _ _ _ _ _ _ _ _ _ _ _ _ _ _ w496 _ _ _ _]
      tunnel: w240 -> [w253 _ _ _ _ _ w420 _ _ _ _ _ _ _ _ _ _ _ _ _ _]
      tunnel: [w252 w297 w399 w404 w413 w417 w418 w427 w437 w444 w456 w468 w475 w478 w482 w490 w495 w517 w519 w523 w534] -> w239
      tunnel: w238 -> [w252 w297 w399 w404 w413 w417 w418 _ _ w444 w456 w468 w475 w478 w482 w490 w495 w517 w519 w523 w534]
      tunnel: w237 -> [w250 _ _ _ _ _ _ _ _ _ _ _ _ _ _ _ _ _ _ _ _]
      event Timeout {
        n139 = event-data() -> ()  [unwired: 1 in, 1 out]
        n140 = local read "Mode"() -> (w255:T4)
        n141 = case shown="\"Basic\"" "Dashboard Tab" {
          tunnel: w258 -> [_ _ w274 _ _]
          tunnel: "/TestMode/Automatic/" ("Name Pattern") -> [_ _ w273 _ _]
          tunnel: T18 [{"Operation"=enum."Clear", "Color Box"=14013909}, {"Operation"=enum."Clear", "Color Box"=14013909}, {"Operation"=enum."Clear", "Color Box"=14013909}, {"Operation"=enum."Clear", "Color Box"=14013909}, {"Operation"=enum."Update", "Color Box"=14013909}, {"Operation"=enum."Update", "Color Box"=16777215}, {"Operation"=enum."Clear", "Color Box"=14013909}, {"Operation"=enum."Clear", "Color Box"=14013909}, {"Operation"=enum."Clear", "Color Box"=14013909}] -> [_ _ w266 _ w290]
          tunnel: w255 -> [_ _ w265 _ w289]
          tunnel: u32[] [15790320, 15790320, 15790320, 15790320, 16777215, 16777215, 15790320, 15790320, 15790320] -> [_ _ _ _ w295]
          tunnel: w253 -> [_ _ _ _ w283]
          tunnel: w250 -> [_ w260 _ _ _]
          frame "Custom", Default {
          }
          frame "Basic" {
            n142 = call <vilib>:"WPI_DashboardUpdateNames.vi"("Controls on Tab"=w260) -> ()  [unwired: 11 in]
          }
          frame "Test" {
            w272 = -2 ("Active Item:Row Number")
            n143 = Index Array(array=w266, index=w265) -> (element=w267:T21)
            n144 = Unbundle(w267) -> ("Operation"=w268:enum16{"Update", "Clear"}, "Color Box"=w269:u32)
            n145 = call <vilib>:"NT Read String.vi"("Name"="/TestMode/TestName") -> ("String"=w263:string)  [unwired: 9 in, 1 out]
            n146 = call <vilib>:"NT Read and Format Entries as Tree.vi"("Operation"=w268, "Name Pattern"=w273, "Tree Refnum"=w274) -> ()  [unwired: 7 in, 2 out]
            n147 = case shown="\"\"" w263 {
              tunnel: "/TestMode/TestProgress" ("Name") -> [w276 _]
              tunnel: "/TestMode/TestProgressText" ("Name") -> [w275 _]
              frame Default {
                n148 = call <vilib>:"NT Read Number.vi"("Name"=w276) -> ("Numeric"=w277:dbl)  [unwired: 9 in, 1 out]
                n149 = call <vilib>:"NT Read String.vi"("Name"=w275) -> ("String"=w278:string)  [unwired: 9 in, 1 out]
                n150 = Bundle("Numeric"=w277, "String"=w278) -> (→"Progress":cluster{"Numeric":dbl, "String":string})  [unwired: 1 in]
              }
              frame "" {
                n151 = property on="Progress" class="Clust (strict)"("Visible"=FALSE) -> ()  [unwired: 2 in, 2 out]
                n152 = local write "Test Name"(u16 0) -> ()
              }
            }
            n153 = property on="Test Tree" class="Tree (strict)"("Active Item Row Number"=w272, "ActiveColNum"=w272, "CellBG"=w269, "Active Item Row Number"=-1 ("Active Item:Row Number"), "CellBG"=u32 5789784 ("Color Box")) -> ()  [unwired: 2 in, 2 out]
          }
          frame "Variables" {
            n154 = control-ref of="Tree"() -> (w282:refnum<vi>)
            n155 = call <vilib>:"NT Read and Format Entries as Tree.vi"("Tree Refnum"=w282) -> ()  [unwired: 9 in, 2 out]
          }
          frame "Commands" {
            w291 = u32 5789784 ("Color Box")
            w292 = T22 {"Row"=-1, "Column"=-2} ("Active Cell:Active Cell")
            w294 = T22 {"Row"=-2, "Column"=-2} ("Active Cell:Active Cell")
            n156 = Index Array(array=w295, index=w289) -> (element=w293:u32)
            n157 = Index Array(array=w290, index=w289) -> (element=w288:T21)
            n158 = Unbundle(w288) -> ("Operation"=w287:enum16{"Update", "Clear"})  [unwired: 1 out]
            n159 = local read "Command Selection"() -> (w286:i32)
            n160 = property on="Command Selection" class="MCListbox (strict)"("ActiveCell"=w294, "CellBG"=w293, "ActiveCell"=w292, "CellBG"=w291) -> ()  [unwired: 2 in, 2 out]
            n161 = call <vilib>:"WPI_DashboardUpdate RPC Info.vi"("Operation"=w287) -> ("update"=w285:bool, "commands"=w284:string[][])  [unwired: 9 in]
            n162 = property on="Command Selection" class="MCListbox (strict)"("ItemNames"=w284) -> ()  [unwired: 2 in, 2 out]
            n163 = property on="Command Params" class="Tbl (strict)"("Active Cell"=w294, "Cell BG Color"=w293, "Active Cell"=w292, "Cell BG Color"=w291) -> ()  [unwired: 2 in, 2 out]
            n164 = call <vilib>:"WPI_DashboardUpdate Command Params.vi"("Update"=w285, "NewVal"=w286, "Commands"=w284, "Param Tbl"=w283) -> ()  [unwired: 7 in, 1 out]
          }
        }
        n165 = call <vilib>:"Connextion Info.vi"() -> ("Connected"=→"NT Connection":bool)  [unwired: 10 in, 1 out]
      }
      event "Test Tree": Value Change {
        # "Show appropriate\ncontrols"
        n166 = event-data() -> ("CtlRef"=w300:refnum<vi>, "NewVal"=w298:string)  [unwired: 1 in]
        n167 = call <vilib>:"WPI_UtilitiesGetTreeIOName.vi"("NewVal"=w298, "TreeControl in"=w300) -> ("I/O Name"=w301:string)  [unwired: 9 in]
        n168 = case shown="\"Camera\"" w301 {
          selector: w301 -> [_ w308 _ w330 w339 _]
          tunnel: w298 -> [_ _ w327 w329 _ w346]
          tunnel: cluster{string[]}[] [{["640x480", "320x240", "160x120"]}, {["Auto", "Fixed indoor", "Fixed outdoor 1", "Fixed outdoor 2", "Fixed fluorescent 1", "Fixed fluorescent 2", "Hold current"]}, {["Auto", "Flicker-free 50 Hz", "Flicker-free 60 Hz", "Hold current"]}, {["None", "Prioritize frame rate", "Prioritize image quality"]}, {["Monochrome", "Color"]}] -> [_ _ _ _ _ w345]
          frame Default {
            w303 = FALSE ("Visible")
            w302 = FALSE ("Visible")
            n169 = property on="Motor" class="Clust (strict)"("Visible"=w302) -> ()  [unwired: 2 in, 2 out]
            n170 = property on="Test Ring" class="Ring (strict)"("Visible"=w302) -> ()  [unwired: 2 in, 2 out]
            n171 = property on="Rev/Fwd" class="Clust (strict)"("Visible"=w303) -> ()  [unwired: 2 in, 2 out]
            n172 = property on="On/Off" class="Bool (strict)"("Visible"=w303) -> ()  [unwired: 2 in, 2 out]
            n173 = property on="Test Slider" class="Slide (strict)"("Visible"=w303) -> ()  [unwired: 2 in, 2 out]
          }
          frame "Analog Out", "Motor", "PWM" {
            w309 = FALSE ("Visible")
            n174 = case shown="\"Analog Out\"" w308 {
              tunnel: [1.0 ("Value") -1.0 ("Value") 0.0 ("Value")] -> w307
              tunnel: [255.0 ("Value") 1.0 ("Value") 5.0 ("Value")] -> w306
              tunnel: [128.0 ("Value") 0.0 ("Value") 0.0 ("Value")] -> w305
              tunnel: [64.0 ("Value") 0.5 ("Value") 1.0 ("Value")] -> w304
              frame "PWM" {
              }
              frame "Motor", Default {
              }
              frame "Analog Out" {
              }
            }
            n175 = property on="Motor" class="Clust (strict)"("Visible"=TRUE) -> ()  [unwired: 2 in, 2 out]
            n176 = property on="Value" class="Slide (strict)"("Value"=w305, "Scale.Minimum"=w307, "Scale.Maximum"=w306, "Scale.Increment"=w304) -> ()  [unwired: 2 in, 2 out]
            n177 = property on="On/Off" class="Bool (strict)"("Visible"=w309) -> ()  [unwired: 2 in, 2 out]
            n178 = property on="Test Slider" class="Slide (strict)"("Visible"=w309) -> ()  [unwired: 2 in, 2 out]
            n179 = property on="Test Ring" class="Ring (strict)"("Visible"=w309) -> ()  [unwired: 2 in, 2 out]
            n180 = property on="Rev/Fwd" class="Clust (strict)"("Visible"=w309) -> ()  [unwired: 2 in, 2 out]
          }
          frame "Servo" {
            w325 = FALSE ("Visible")
            n181 = call <vilib>:"NT Read Number.vi"("Name"=w327) -> ("Numeric"=w326:dbl)  [unwired: 9 in, 1 out]
            n182 = property on="Test Slider" class="Slide (strict)"("Visible"=TRUE, "Scale.Maximum"=170.0 ("Scale.Range:Maximum")) -> ()  [unwired: 2 in, 2 out]
            n183 = local write "Test Slider"(w326) -> ()
            n184 = property on="Motor" class="Clust (strict)"("Visible"=w325) -> ()  [unwired: 2 in, 2 out]
            n185 = property on="Rev/Fwd" class="Clust (strict)"("Visible"=w325) -> ()  [unwired: 2 in, 2 out]
            n186 = property on="On/Off" class="Bool (strict)"("Visible"=w325) -> ()  [unwired: 2 in, 2 out]
            n187 = property on="Test Ring" class="Ring (strict)"("Visible"=w325) -> ()  [unwired: 2 in, 2 out]
          }
          frame "Relay", "Solenoid" {
            w328 = FALSE ("Visible")
            n188 = property on="Motor" class="Clust (strict)"("Visible"=w328) -> ()  [unwired: 2 in, 2 out]
            n189 = property on="Test Slider" class="Slide (strict)"("Visible"=w328) -> ()  [unwired: 2 in, 2 out]
            n190 = Search and Replace String(input string=w329, search string="/Value  **", replace string="/Direction") -> (result string=w335:string)  [unwired: 5 in, 3 out]
            n191 = property on="Test Ring" class="Ring (strict)"("Visible"=w328) -> ()  [unwired: 2 in, 2 out]
            n192 = call <vilib>:"NT Read String.vi"("Name"=w335) -> ("String"=w333:string)  [unwired: 9 in, 1 out]
            n193 = Equal?(x="Both directions", y=w333) -> (x = y?=w331:bool)
            n194 = Not(x=w331) -> (.not. x?=w332:bool)
            n195 = property on="Rev/Fwd" class="Clust (strict)"("Visible"=w331) -> ()  [unwired: 2 in, 2 out]
            n196 = property on="On/Off" class="Bool (strict)"("Visible"=w332, "Caption.Text"=w330) -> ()  [unwired: 2 in, 2 out]
          }
          frame "Compressor", "Digital Out" {
            w338 = FALSE ("Visible")
            # "Get direction and finish"
            n197 = property on="Motor" class="Clust (strict)"("Visible"=w338) -> ()  [unwired: 2 in, 2 out]
            n198 = property on="Test Slider" class="Slide (strict)"("Visible"=w338) -> ()  [unwired: 2 in, 2 out]
            n199 = property on="Test Ring" class="Ring (strict)"("Visible"=w338) -> ()  [unwired: 2 in, 2 out]
            n200 = property on="On/Off" class="Bool (strict)"("Visible"=TRUE, "Caption.Text"=w339) -> ()  [unwired: 2 in, 2 out]
            n201 = property on="Rev/Fwd" class="Clust (strict)"("Visible"=FALSE) -> ()  [unwired: 2 in, 2 out]
          }
          frame "Camera" {
            n202 = call <vilib>:"Get Last Path Segment.vi"("String in"=w346) -> ("String out"=w347:string)  [unwired: 10 in]
            n203 = property on="On/Off" class="Bool (strict)"("Visible"=FALSE) -> ()  [unwired: 2 in, 2 out]
            n204 = property on="Motor" class="Clust (strict)"("Visible"=FALSE) -> ()  [unwired: 2 in, 2 out]
            n205 = property on="Rev/Fwd" class="Clust (strict)"("Visible"=FALSE) -> ()  [unwired: 2 in, 2 out]
            n206 = case shown="\"White Balance  **\"" w347 {
              tunnel: w346 -> [w353 w362 w371 w380 w389 _ w395]
              tunnel: w345 -> [w351 w359 w368 w377 w386 _ _]
              frame "Size  **" {
                n207 = Index Array(array=w351) -> (element=w350:cluster{string[]})  [unwired: 1 in]
                n208 = call <vilib>:"NT Read String.vi"("Name"=w353) -> ("String"=w352:string)  [unwired: 9 in, 1 out]
                n209 = Unbundle(w350) -> (w348:string[])
                n210 = Match First String(2:w348, 3:w352) -> (0:w349:i32)  [unwired: 1 out]
                n211 = property on="Test Ring" class="Ring (strict)"("Value"=w349, "Strings []"=w348) -> ()  [unwired: 2 in, 2 out]
                n212 = property on="Test Ring" class="Ring (strict)"("Visible"=TRUE) -> ()  [unwired: 2 in, 2 out]
                n213 = property on="Test Slider" class="Slide (strict)"("Visible"=FALSE) -> ()  [unwired: 2 in, 2 out]
              }
              frame "White Balance  **" {
                n214 = Index Array(array=w359, index=1) -> (element=w360:cluster{string[]})
                n215 = call <vilib>:"NT Read String.vi"("Name"=w362) -> ("String"=w361:string)  [unwired: 9 in, 1 out]
                n216 = Unbundle(w360) -> (w357:string[])
                n217 = Match First String(2:w357, 3:w361) -> (0:w356:i32)  [unwired: 1 out]
                n218 = property on="Test Ring" class="Ring (strict)"("Value"=w356, "Strings []"=w357) -> ()  [unwired: 2 in, 2 out]
                n219 = property on="Test Ring" class="Ring (strict)"("Visible"=TRUE) -> ()  [unwired: 2 in, 2 out]
                n220 = property on="Test Slider" class="Slide (strict)"("Visible"=FALSE) -> ()  [unwired: 2 in, 2 out]
              }
              frame "Exposure  **" {
                n221 = Index Array(array=w368, index=2) -> (element=w369:cluster{string[]})
                n222 = call <vilib>:"NT Read String.vi"("Name"=w371) -> ("String"=w370:string)  [unwired: 9 in, 1 out]
                n223 = Unbundle(w369) -> (w365:string[])
                n224 = Match First String(2:w365, 3:w370) -> (0:w366:i32)  [unwired: 1 out]
                n225 = property on="Test Ring" class="Ring (strict)"("Value"=w366, "Strings []"=w365) -> ()  [unwired: 2 in, 2 out]
                n226 = property on="Test Ring" class="Ring (strict)"("Visible"=TRUE) -> ()  [unwired: 2 in, 2 out]
                n227 = property on="Test Slider" class="Slide (strict)"("Visible"=FALSE) -> ()  [unwired: 2 in, 2 out]
              }
              frame "Exposure Priority  **" {
                n228 = Index Array(array=w377, index=3) -> (element=w378:cluster{string[]})
                n229 = call <vilib>:"NT Read String.vi"("Name"=w380) -> ("String"=w379:string)  [unwired: 9 in, 1 out]
                n230 = Unbundle(w378) -> (w374:string[])
                n231 = Match First String(2:w374, 3:w379) -> (0:w375:i32)  [unwired: 1 out]
                n232 = property on="Test Ring" class="Ring (strict)"("Value"=w375, "Strings []"=w374) -> ()  [unwired: 2 in, 2 out]
                n233 = property on="Test Ring" class="Ring (strict)"("Visible"=TRUE) -> ()  [unwired: 2 in, 2 out]
                n234 = property on="Test Slider" class="Slide (strict)"("Visible"=FALSE) -> ()  [unwired: 2 in, 2 out]
              }
              frame "Color Enable  **" {
                n235 = Index Array(array=w386, index=4) -> (element=w387:cluster{string[]})
                n236 = call <vilib>:"NT Read String.vi"("Name"=w389) -> ("String"=w388:string)  [unwired: 9 in, 1 out]
                n237 = Unbundle(w387) -> (w383:string[])
                n238 = Match First String(2:w383, 3:w388) -> (0:w384:i32)  [unwired: 1 out]
                n239 = property on="Test Ring" class="Ring (strict)"("Value"=w384, "Strings []"=w383) -> ()  [unwired: 2 in, 2 out]
                n240 = property on="Test Ring" class="Ring (strict)"("Visible"=TRUE) -> ()  [unwired: 2 in, 2 out]
                n241 = property on="Test Slider" class="Slide (strict)"("Visible"=FALSE) -> ()  [unwired: 2 in, 2 out]
              }
              frame Default {
                n242 = property on="Test Ring" class="Ring (strict)"("Visible"=FALSE) -> ()  [unwired: 2 in, 2 out]
                n243 = property on="Test Slider" class="Slide (strict)"("Visible"=FALSE) -> ()  [unwired: 2 in, 2 out]
              }
              frame "Brightness  **", "Color Level  **", "Compression  **", "FPS  **", "Sharpness  **" {
                n244 = call <vilib>:"NT Read Number.vi"("Name"=w395) -> ("Numeric"=w394:dbl)  [unwired: 9 in, 1 out]
                n245 = local write "Test Slider"(w394) -> ()
                n246 = property on="Test Slider" class="Slide (strict)"("Visible"=TRUE, "Scale.Maximum"=100.0 ("Scale.Range:Maximum")) -> ()  [unwired: 2 in, 2 out]
                n247 = property on="Test Ring" class="Ring (strict)"("Visible"=FALSE) -> ()  [unwired: 2 in, 2 out]
              }
            }
          }
        }
        n248 = property on="Progress" class="Clust (strict)"("Visible"=FALSE) -> ()  [unwired: 2 in, 2 out]
      }
      event "Test Name": Mouse Enter {
        # "Populate the ring with the list of tests"
        n249 = event-data() -> ()  [unwired: 1 in, 1 out]
        n250 = call <vilib>:"NT Read String Array.vi"("Name"="/TestMode/TestList") -> ("String Array"=w403:string[])  [unwired: 9 in, 1 out]
        n251 = Build Array (concatenate)("Select the test to run...", w403) -> (w402:string[])
        n252 = property on="Test Name" class="Ring (strict)"("Strings []"=w402) -> ()  [unwired: 2 in, 2 out]
      }
      event "Test Name": Value Change {
        w405 = FALSE ("Visible")
        # "Tell the robot the test name to run"
        n253 = event-data() -> ("NewVal"=w409:u16)  [unwired: 1 in]
        n254 = property on="Test Name" class="Ring (strict)"() -> ("Strings []"=w410:string[])  [unwired: 2 in, 2 out]
        n255 = local write "Progress"(T6 {"Test Progress"=0, "Test Progress Text"=""} ("Progress")) -> ()
        n256 = Index Array(array=w410, index=w409) -> (element=w408:string)
        n257 = call <vilib>:"NT Write String.vi"("String"=w408, "Name"="/TestMode/TestName") -> ()  [unwired: 9 in, 1 out]
        n258 = property on="Progress" class="Clust (strict)"("Visible"=TRUE) -> ()  [unwired: 2 in, 2 out]
        n259 = property on="Motor" class="Clust (strict)"("Visible"=w405) -> ()  [unwired: 2 in, 2 out]
        n260 = property on="Test Slider" class="Slide (strict)"("Visible"=w405) -> ()  [unwired: 2 in, 2 out]
        n261 = property on="On/Off" class="Bool (strict)"("Visible"=w405) -> ()  [unwired: 2 in, 2 out]
        n262 = property on="Rev/Fwd" class="Clust (strict)"("Visible"=w405) -> ()  [unwired: 2 in, 2 out]
        n263 = property on="Test Ring" class="Ring (strict)"("Visible"=w405) -> ()  [unwired: 2 in, 2 out]
      }
      event "Select Auto": Mouse Enter {
        # "Populate the combo box with the list of autonomous options"
        n264 = event-data() -> ()  [unwired: 1 in, 1 out]
        n265 = call <vilib>:"NT Read String Array.vi"("Name"="Auto List") -> ("String Array"=w412:string[])  [unwired: 9 in, 1 out]
        n266 = property on="Select Auto" class="CmbBox"("Strings[]"=w412) -> ()  [unwired: 2 in, 2 out]
      }
      event "Select Auto": Value Change {
        # "User modified the Auto Selection. Write to NT variable so robot knows."
        n267 = event-data() -> ("NewVal"=w415:string)  [unwired: 1 in]
        n268 = call <vilib>:"NT Write String.vi"("String"=w415, "Name"="Auto Selector") -> ()  [unwired: 9 in, 1 out]
      }
      event "Command Selection": Value Change {
        # "Get the params and show in table"
        n269 = event-data() -> ("NewVal"=w421:i32)  [unwired: 1 in]
        n270 = property on="Command Selection" class="MCListbox (strict)"() -> ("ItemNames"=w419:string[][])  [unwired: 2 in, 2 out]
        n271 = call <vilib>:"WPI_DashboardUpdate Command Params.vi"("NewVal"=w421, "Commands"=w419, "Param Tbl"=w420) -> ()  [unwired: 8 in, 1 out]
      }
      event "Execute Command": Value Change {
        # "Started one, Unique ID holds\nresponse"
        n272 = event-data() -> ()  [unwired: 1 in, 1 out]
        n273 = property on="Command Selection" class="MCListbox (strict)"() -> ("ItemNames"=w432:string[][])  [unwired: 2 in, 2 out]
        n274 = Index Array(array=w432, index (row)="Command Selection", index (col)=0) -> (element=w430:string)
        n275 = call <vilib>:"Invoke Commands.vi"("Command Params"="Command Params", "Function Name"=w430) -> ("Params"=w426:u8, "Started"=w425:bool)  [unwired: 7 in, 1 out]
        n276 = Array Subset(array="Command Params", length (row)=w426) -> (w427:string[][])  [unwired: 3 in]
        n277 = Select(t="Executing" ("Cmd Status"), s=w425, f="" ("Cmd Status")) -> (s? t:f=→"Cmd Status":string)
      }
      event "Command Selection": Double Click {
        n278 = event-data() -> ("Row"=w440:i32)  [unwired: 1 in]
        n279 = property on="Command Selection" class="MCListbox (strict)"() -> ("ItemNames"=w443:string[][])  [unwired: 2 in, 2 out]
        n280 = local read "Command Params"() -> (w439:string[][])
        n281 = Index Array(array=w443, index (row)=w440, index (col)=0) -> (element=w441:string)
        n282 = call <vilib>:"Invoke Commands.vi"("Command Params"=w439, "Function Name"=w441) -> ("Params"=w438:u8, "Started"=w433:bool)  [unwired: 7 in, 1 out]
        n283 = Array Subset(array=w439, length (row)=w438) -> (w437:string[][])  [unwired: 3 in]
        n284 = Select(t="Executing" ("Cmd Status"), s=w433, f="" ("Cmd Status")) -> (s? t:f=w434:string)
        n285 = local write "Cmd Status"(w434) -> ()
      }
      event "CheckList": Double Click {
        # "Shift clears all"
        # "Update symbols on the listbox"
        n286 = event-data() -> ("PlatMods.Shift"=w445:bool, "Row"=w447:i32)  [unwired: 1 in]
        n287 = case shown="True" w445 {
          tunnel: w447 -> [w451 _]
          tunnel: 1 -> [w450 _]
          frame False {
            n288 = property on="CheckList" class="LstBox (strict)"() -> ("Item Symbols"=w449:i32[])  [unwired: 2 in, 2 out]
            n289 = Replace Array Subset(array=w449, new element=w450, index=w451) -> (w448:i32[])
            n290 = property on="CheckList" class="LstBox (strict)"("Item Symbols"=w448) -> ()  [unwired: 2 in, 2 out]
          }
          frame True {
            w452 = 0 ("Top Row")
            n291 = property on="CheckList" class="LstBox (strict)"() -> ("Number of Rows"=w454:u32)  [unwired: 2 in, 2 out]
            n292 = Initialize Array(0, w454) -> (w453:i32[])
            n293 = property on="CheckList" class="LstBox (strict)"("Top Row"=w452, "Value"=w452, "Item Symbols"=w453) -> ()  [unwired: 2 in, 2 out]
          }
        }
      }
      event "CheckList": Key Down {
        # "Update symbols on the listbox\nLeft and right keys check and uncheck"
        n294 = event-data() -> ("VKey"=w458:T19)  [unwired: 1 in]
        n295 = case shown="\"Left\", \"Right\"" w458 {
          selector: w458 -> [w463 _]
          tunnel: eventvkey."Left" ("VKey") -> [w461 _]
          frame "Left", "Right" {
            n296 = Equal?(x=w461, y=w463) -> (x = y?=w462:bool)
            n297 = Select(t=0, s=w462, f=1) -> (s? t:f=w464:i32)
            n298 = property on="CheckList" class="LstBox (strict)"() -> ("Item Symbols"=w467:i32[])  [unwired: 2 in, 2 out]
            n299 = Replace Array Subset(array=w467, new element=w464, index="CheckList") -> (w466:i32[])
            n300 = property on="CheckList" class="LstBox (strict)"("Item Symbols"=w466) -> ()  [unwired: 2 in, 2 out]
          }
          frame Default {
          }
        }
      }
      event "Motor.Enable": Value Change {
        # "When the test mode otor enable helper is set, update that\ntree row item's value"
        n301 = event-data() -> ("NewVal"=w473:bool)  [unwired: 1 in]
        n302 = Unbundle("Motor") -> ("Value"=w472:dbl)  [unwired: 1 out]
        n303 = Select(t=w472, s=w473, f=0.0) -> (s? t:f=w470:dbl)
        n304 = call <vilib>:"NT Write Number.vi"("Numeric"=w470, "Name"=w469) -> ()  [unwired: 9 in, 1 out]
      }
      event "Test Slider": Value Change {
        # "When the test mode slider helper is set, update that\ntree row item's value"
        n305 = event-data() -> ("NewVal"=w476:dbl)  [unwired: 1 in]
        n306 = call <vilib>:"NT Write Number.vi"("Numeric"=w476, "Name"=w477) -> ()  [unwired: 9 in, 1 out]
      }
      event "On/Off": Value Change {
        # "When the test mode on/off helper value is set, update that\ntree row item's value"
        n307 = event-data() -> ("NewVal"=w481:bool)  [unwired: 1 in]
        n308 = Boolean To (0,1)(Boolean=w481) -> (0, 1=w480:i16)
        n309 = call <vilib>:"NT Write Number.vi"("Numeric"=w480, "Name"=w479) -> ()  [unwired: 9 in, 1 out]
      }
      event "Rev/Fwd": Value Change {
        # "When the test mode helper value for relays is set, update that\ntree row item's value"
        n310 = event-data() -> ("NewVal.Forward"=w489:bool, "NewVal.Reverse"=w488:bool)  [unwired: 1 in]
        n311 = Boolean To (0,1)(Boolean=w489) -> (0, 1=w485:i16)
        n312 = Boolean To (0,1)(Boolean=w488) -> (0, 1=w487:i16)
        n313 = Negate(x=w487) -> (-x=w486:i16)
        n314 = Add(x=w485, y=w486) -> (x+y=w484:i16)
        n315 = call <vilib>:"NT Write Number.vi"("Numeric"=w484, "Name"=w483) -> ()  [unwired: 9 in, 1 out]
      }
      event "Test Ring": Value Change {
        # "When a test mode helper value is selected from the ring,\nset the tree item's variable to the string value"
        n316 = event-data() -> ("NewVal"=w493:u16)  [unwired: 1 in]
        n317 = property on="Test Ring" class="Ring (strict)"() -> ("Strings []"=w494:string[])  [unwired: 2 in, 2 out]
        n318 = Index Array(array=w494, index=w493) -> (element=w492:string)
        n319 = call <vilib>:"NT Write String.vi"("String"=w492, "Name"=w491) -> ()  [unwired: 9 in, 1 out]
      }
      event "Rec Mode": Value Change {
        # "Update globals for recording mode and path to read log from.\nClear when logging and let NetworkTables set path for vision to\nuse."
        n320 = event-data() -> ("NewVal"=w505:enum32{"Stop", "Record", "Playback"})  [unwired: 1 in]
        n321 = global write "WPI_DashboardLogging Global.vi" "Logging Filename"(path "") -> ()
        n322 = global write "WPI_DashboardLogging Global.vi" "Recording"(w505) -> ()
        n323 = case shown="\"Playback\"" w505 {
          tunnel: w504 -> [_ w507 w516]
          tunnel: [_ _ w515] -> w502
          tunnel: [_ _ w514] -> _
          tunnel: w500 -> [_ _ w512]
          tunnel: cluster{i32, i32} {-250, 170} -> [_ _ w511]
          tunnel: [_ _ T20 {"Image Size"=TRUE, "Image Type"=TRUE, "Pixel Value"=TRUE, "ROI Information"=TRUE, "Zoom Factor"=FALSE} ("Image Information Shown:All Elements")] -> w498
          tunnel: [_ _ TRUE ("Zoom Factor")] -> w497
          tunnel: w496 -> [_ _ w508]
          frame Default {
          }
          frame "Stop", "Record" {
            # "Place Window too"
            n324 = invoke class="VI" method="FP.Close"(reference=w507) -> (reference out=w506:refnum<vi>)  [unwired: 2 in, 2 out]
            n325 = invoke class="VI" method="Abort VI"(reference=w506) -> ()  [unwired: 2 in, 3 out]
          }
          frame "Playback" {
            n326 = call "Open Playback Panel.vi"("Offset"=w511, "DB VI Ref"=w512, "Playback in"=w516) -> ("Playback out"=w513:refnum<vi>)  [unwired: 8 in]
            n327 = register-events(w513, w508) -> (reference out=w515:refnum<event-registration>, error out=w514:errorcluster)  [unwired: 2 in]
          }
        }
        n328 = property on="Camera Image" class="ImageControl"("Image Information Shown"=w498, "Image Information Visible"=w497) -> ()  [unwired: 2 in, 2 out]
        n329 = call <vilib>:"WPI_DashboardNT Log FieldName Cache.vi"("Operation"=enum16{"Lookup/Add", "Index", "Clear"}."Clear") -> ()  [unwired: 8 in, 3 out]
      }
      event Panel Close {
        w518 = enum32{"Stop", "Record", "Playback"}."Stop" ("Rec Mode")
        # "Playback window has been closed, abort"
        n330 = event-data() -> ()  [unwired: 1 in, 4 out]
        n331 = local write "Rec Mode"(w518) -> ()
        n332 = global write "WPI_DashboardLogging Global.vi" "Recording"(w518) -> ()
      }
      event Panel Close {
        # "Abort playback window and ourself"
        n333 = event-data() -> ()  [unwired: 1 in, 4 out]
        n334 = invoke class="VI" method="FP.Close"(reference=w522) -> (reference out=w521:refnum<vi>)  [unwired: 2 in, 2 out]
        n335 = invoke class="VI" method="Abort VI"(reference=w521) -> (error out=w520:errorcluster)  [unwired: 2 in, 2 out]
        n336 = invoke class="VI" method="Abort VI"(error in=w520) -> ()  [unwired: 2 in, 3 out]
      }
      event User Event {
        n337 = event-data() -> ("IDs"=w529:cluster{"RPC field ID":u16, "Unique ID":u16}, "String"=w528:string)  [unwired: 1 in]
        n338 = Bundle("IDs"=w529, "String"=w528) -> (w527:T8)  [unwired: 1 in]
        n339 = call <vilib>:"Retrieve RPC Response.vi"("RPC Response"=w527) -> ("Output"=w525:string[][])  [unwired: 10 in]
        n340 = Build Array (concatenate)(w523, w525) -> (w524:string[][])
        n341 = local write "Command Params"(w524) -> ()
        n342 = local write "Cmd Status"("" ("Cmd Status")) -> ()
      }
      event "Tree": Double Click {
        n343 = event-data() -> ("PlatMods"=w533:T23, "Tag"=w532:string)  [unwired: 1 in]
        n344 = Unbundle(w533) -> ("Shift"=w531:bool)  [unwired: 4 out]
        n345 = Not(x=w531) -> (.not. x?=w530:bool)
        n346 = call <vilib>:"NT Update Persistence.vi"("Persistence"=w530, "Name"=w532) -> ()  [unwired: 9 in, 1 out]
      }
    }
  }
  n347 = while {
    tunnel: w64 -> [w536]
    i -> [w539]
    stop <- FALSE stop-if-true
    n348 = Wait (ms)(milliseconds to wait=u32 100) -> ()  [unwired: 1 out]
    n349 = case shown="\"Playback\"" "Rec Mode" {
      tunnel: w539 -> [_ _ w554]
      tunnel: [u32 2829099 ("Base Color") u32 11141120 ("Target Color") w543] -> w535
      frame "Stop", Default {
        # "Reset the color, extra updates don't cost much"
      }
      frame "Record" {
      }
      frame "Playback" {
        # "Playback"
        n350 = Quotient & Remainder(x=w554, y=u32 50 ("milliseconds to wait")) -> (x-y*floor(x/y)=w550:u32)  [unwired: 1 out]
        n351 = Divide(x=w550, y=u32 50 ("milliseconds to wait")) -> (x/y=w547:dbl)
        n352 = Multiply(x=6.283185307179586, y=w547) -> (x*y=w552:dbl)
        n353 = Sine(x=w552) -> (sin(x)=w551:dbl)
        n354 = Absolute Value(x=w551) -> (abs(x)=w544:dbl)
        n355 = call "Interpolate RGB Color.vi"("Proportion"=w544, "Target Color"=u32 30976, "Base Color"=u32 2829099) -> ("Result Color"=w543:u32)  [unwired: 8 in]
      }
    }
    n356 = property class="Pane"(reference=w536, "PaneColor"=w535) -> ()  [unwired: 1 in, 2 out]
  }
  n357 = local write "Dashboard Tab"(T2."Drive" ("Dashboard Tab")) -> ()
  n358 = property on="On/Off" class="Bool (strict)"("Visible"=w33) -> ()  [unwired: 2 in, 2 out]
  n359 = property on="Motor" class="Clust (strict)"("Visible"=w33) -> ()  [unwired: 2 in, 2 out]
  n360 = property on="Progress" class="Clust (strict)"("Visible"=w33) -> ()  [unwired: 2 in, 2 out]
  n361 = property on="Test Ring" class="Ring (strict)"("Visible"=w33) -> ()  [unwired: 2 in, 2 out]
  n362 = property on="Rev/Fwd" class="Clust (strict)"("Visible"=w33) -> ()  [unwired: 2 in, 2 out]
  n363 = local write "Command Selection"(u16 0 ("milliseconds to wait")) -> ()
  n364 = local write "Command Params"(string[][] [] ("Command Params")) -> ()
  n365 = global write "WPI_DashboardLogging Global.vi" "Recording"(w58) -> ()
  n366 = local write "Rec Mode"(w58) -> ()
  n367 = while {
    tunnel: u16 1741 ("timeout ms (25000)") -> [w556]
    stop <- FALSE stop-if-true
    n368 = TCP Create Listener(10:w556) -> (0:w555:errorcluster, 3:w557:refnum<k5>)  [unwired: 4 in, 1 out]
    n369 = case shown="No Error" w555 {
      selector: w555 -> [w559 _]
      tunnel: w557 -> [w560 _]
      frame No Error {
        n370 = while {
          tunnel: w560 -> [w563]
          tunnel: w559 -> [w562]
          stop <- FALSE stop-if-true
          n371 = TCP Wait On Listener(8:w562, 11:w563) -> (0:w564:errorcluster, 4:w565:refnum<k5>)  [unwired: 2 in, 3 out]
          n372 = local write "TCP"(w565) -> ()
          n373 = case shown="No Error" w564 {
            frame No Error {
            }
            frame Error {
              n374 = Wait (ms)(milliseconds to wait=u32 1000) -> ()  [unwired: 1 out]
            }
          }
        }
      }
      frame Error {
        n375 = Wait (ms)(milliseconds to wait=u32 1000) -> ()  [unwired: 1 out]
      }
    }
  }
  n376 = call <vilib>:"NT Write String.vi"("String"="Select Auto", "Name"="Auto Selector") -> ()  [unwired: 9 in, 1 out]
